vi "SlopeOfLine.vi"() -> ()   [LabVIEW 2025]
panel:
  out "Numeric":dbl
  in  "y2":dbl
  in  "y1":dbl
  in  "x2":dbl
  in  "x1":dbl
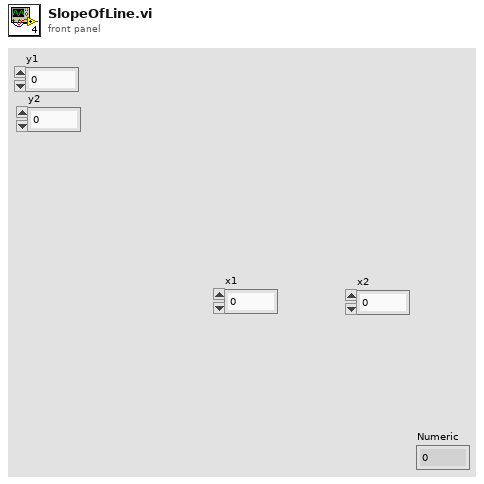
[diagram p1: front panel]
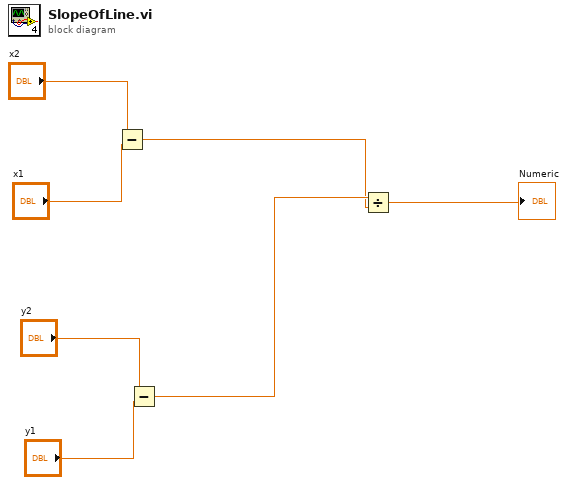
[diagram p0: block diagram]
diagram:
  n1 = Subtract(x="x2", y="x1") -> (x-y=w2:dbl)
  n2 = Subtract(x="y2", y="y1") -> (x-y=w3:dbl)
  n3 = Divide(x=w3, y=w2) -> (x/y=→"Numeric":dbl)
